vi "Initialize.vi"(8 "error in":errorcluster, 10 "parameters":variant, 11 "node in":refnum<class "SystemLink File editor node.lvclass">) -> (0 "error out":errorcluster, 2 "summary":T2[](array[typedef]), 3 "data value reference":T1)   [LabVIEW 2015, in "SystemLink File editor node.lvclass"]
doc: "Initializes the data of a node to its default state.\nThe object is not created inside of this VI, because it is created from a File depending on user selection.\nCopyright 2017 National Instruments Corporation\n\nLicensed under the Apache License, Version 2.0 (the \"License\"); you may not use this file except in compliance with the License. You may obtain a copy of the License at http://www.apache.org/licenses/LICENSE-2.0\nUnless required by applicable law or agreed to in writing, software distributed under the License is distributed on an \"AS IS\" BASIS, WITHOUT WARRANTIES OR CONDITIONS OF ANY KIND, either express or implied. See the License for the specific language governing permissions and limitations under the License."
uses:
  SystemLink File editor node.lvclass
  <vilib>/NI/Configuration Framework/Node/Summary.ctl
  <vilib>/NI/Configuration Framework/Node/NodeRef.ctl
  <vilib>/NI/Configuration Framework/Node/NISE_CEF_Node.lvclass
  module/configuration/SystemLink File configuration.lvclass
  <vilib>/NI/Tag Bus/tag/Data Type.ctl
  <vilib>/NI/Tag Bus Module Framework/channel/channel classification.ctl
  <vilib>/NI/Configuration Framework/serializable configuration/NISE_CEF_serializable configuration.lvclass
  <vilib>/NI/DCAF/Tag Editor Core/Configuration Editor/Classes/Module editor node/module editor node.lvclass
  <vilib>/NI/Tag Bus Module Framework/channel/TBM channel.lvclass
  <vilib>/NI/Tag Bus/tag/tag descriptor.lvclass
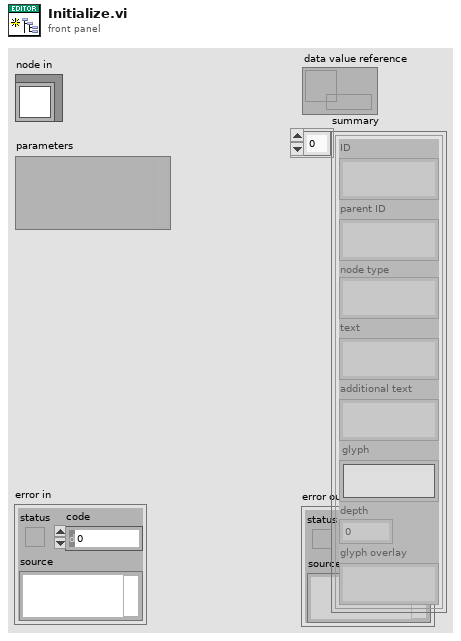
[diagram p1: front panel]
types:
  T1 = typedef "NISE_CEF_Node.lvclass/NodeRef.ctl" = refnum<data-value>
  T2 = typedef "NISE_CEF_Node.lvclass/Summary.ctl" = cluster{"ID":string, "parent ID":string, "node type":string, "text":string, "additional text":string, "glyph":string, "depth":i32, "glyph overlay":string}
  T3 = typedef "TBM channel.lvclass/channel classification.ctl" = enum16{"input data", "output data", "processing parameter", "processing result"}
  T4 = typedef "tag bus.lvlib/tag descriptor.lvclass/Data Type.ctl" = enum16{"Double", "Single", "I64", "I32", "I16", "I8", "U64", "U32", "U16", "U8", "Boolean", "String", "Array of Double", "Array of Single", "Array of I64", "Array of I32", "Array of I16", "Array of I8", "Array of U64", "Array of U32", "Array of U16", "Array of U8", "Array of Boolean", "Array of String"}
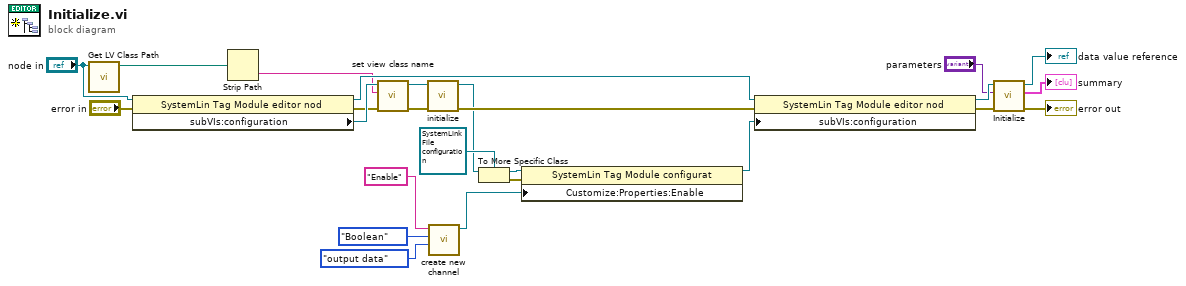
[diagram p0: block diagram]
diagram:
  n1 = call <vilib>:"Get LV Class Path.vi"("object"="node in") -> ("class path"=w17:path)  [unwired: 9 in, 1 out]
  n2 = property class="SystemLin Tag Module editor nod"(reference="node in", error in="error in") -> (reference out=w23:refnum<class "SystemLink File editor node.lvclass">, error out=w18:errorcluster, "subVIs:configuration"=w21:refnum<class "NISE_CEF_serializable configuration.lvclass">)
  n3 = Strip Path(path=w17) -> (name=w16:string)  [unwired: 1 out]
  n4 = call <vilib>:"set view class name.vi"("error in"=w18, "view class"=w16, "configuration in"=w21) -> ("error out"=w19:errorcluster, "configuration out"=w20:refnum<class "NISE_CEF_serializable configuration.lvclass">)  [unwired: 7 in]
  n5 = call <vilib>:"initialize.vi"("error in"=w19, "configuration in"=w20) -> ("error out"=w22:errorcluster, "configuration out"=w7:refnum<class "NISE_CEF_serializable configuration.lvclass">)  [unwired: 7 in, 1 out]
  n6 = call <vilib>:"create new channel.vi"("channel classification"=channel_classification."output data", "data type"=Data_Type."Boolean", "channel name"="Enable") -> ("channel"=w1:refnum<class "TBM channel.lvclass">)  [unwired: 8 in]
  n7 = To More Specific Class(target class=refnum<class "SystemLink File configuration.lvclass"> refnum ("SystemLin Tag Module configuration"), reference=w7) -> (specific class reference=w5:refnum<class "SystemLink File configuration.lvclass">, error out=w6:errorcluster)  [unwired: 1 in]
  n8 = property class="SystemLin Tag Module configurat"(reference=w5, error in=w6, "Customize:Properties:Enable"=w1) -> (reference out=w9:refnum<class "SystemLink File configuration.lvclass">)  [unwired: 1 out]
  n9 = property class="SystemLin Tag Module editor nod"(reference=w23, error in=w22, "subVIs:configuration"=w9) -> (reference out=w24:refnum<class "SystemLink File editor node.lvclass">, error out=w25:errorcluster)
  n10 = call-parent <vilib>:"Initialize.vi"("error in"=w25, "parameters"="parameters", "node in"=w24) -> ("error out"=→"error out":errorcluster, "summary"=→"summary":T2[], "data value reference"=→"data value reference":T1)  [unwired: 6 in]
